vi "Update DO Bit with Index_PrivateData.vi"(8 "error in (no error)":errorcluster, 9 "Value":bool, 10 "index":i32, 11 "IO in":refnum<class "IO.lvclass">) -> (0 "error out":errorcluster, 2 "DO Bits Value":bool[](array[boolean]), 3 "IO out":refnum<class "IO.lvclass">)   [LabVIEW 2022 SP3, in "IO.lvclass"]
uses:
  IO.lvclass
  IO.lvclass/IO.ctl
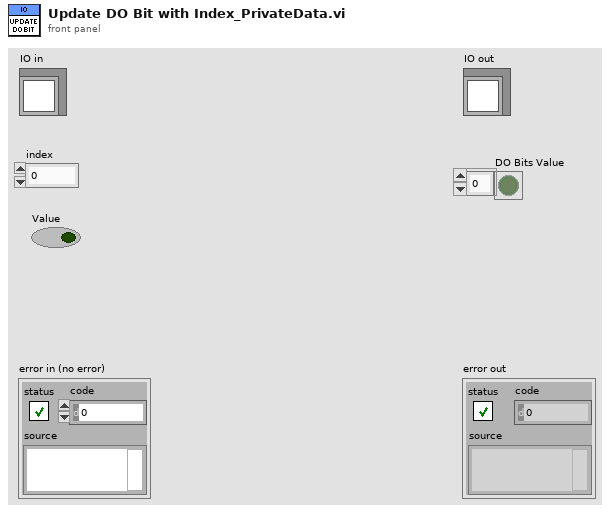
[diagram p1: front panel]
types:
  T1 = typedef "IO.lvclass/Private Data.ctl" = cluster{"UserEvents":T2, "All Dependencies":cluster{"Class References":refnum<class>[], "Class Names":string[]}, "Status":T3}
  T2 = typedef "IO.lvclass/UserEvents.ctl" = cluster{"API Incoming Event":refnum<user-event>, "API Executed Event":refnum<user-event>, "API Return Event":refnum<user-event>, "Status Changed Event":refnum<user-event>}
  T3 = typedef "IO.lvclass/Status Cluster.ctl" = cluster{"DO Bits Value":bool[], "Device Data":variant, "Ordered DI Channels":T4[], "Ordered DO Channels":T5[]}
  T4 = typedef "IO.lvclass/DI Channel Names.ctl" = enum16{"None", "SW - Ink Valve - R1", "SW - Ink Valve - R2", "SW - Ink Valve - R3", "SW - Ink Valve - R4", "SW - Ink Valve - R5", "SW - Ink Valve - R6", "SW - COVER INPUT SIDE", "SW - COVER OUTPUT SIDE", "SW - Purge - R1", "SW - Purge - R2", "SW - Purge - R3", "SW - Purge - R4", "SW - Purge - R5", "SW - Purge - R6"}
  T5 = typedef "IO.lvclass/DO Channel Names.ctl" = enum16{"None", "Meniscus Valve Open - R1", "Meniscus Valve Open - R2", "Meniscus Valve Open - R3", "Meniscus Valve Open - R4", "Meniscus Valve Open - R5", "Meniscus Valve Open - R6", "Ink Flow Valve Open - R1", "Ink Flow Valve Open - R2", "Ink Flow Valve Open - R3", "Ink Flow Valve Open - R4", "Ink Flow Valve Open - R5", "Ink Flow Valve Open - R6", "SW_LED - Ink Valve - R1", "SW_LED - Ink Valve - R2", "SW_LED - Ink Valve - R3", "Recirc Pump On - R1", "Recirc Pump On - R2", "Recirc Pump On - R3", "Recirc Pump On - R4", "Recirc Pump On - R5", "Recirc Pump On - R6", "SW_LED - Ink Valve - R4", "SW_LED - Ink Valve - R5", "SW_LED - Ink Valve - R6"}
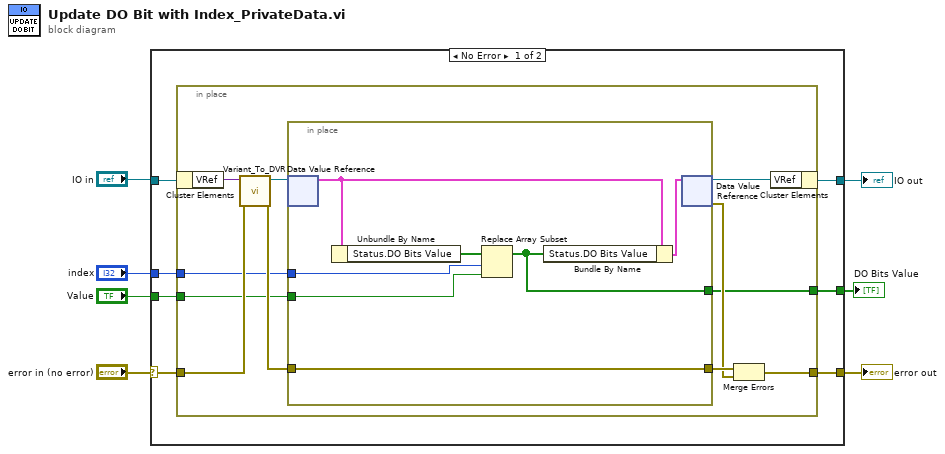
[diagram p0: block diagram]
diagram:
  n1 = case shown="No Error" "error in (no error)" {
    selector: "error in (no error)" -> [w11 w34]
    tunnel: [w13 w34] -> w5
    tunnel: [w14 w33] -> w4
    tunnel: "IO in" -> [w12 w33]
    tunnel: "index" -> [w10 _]
    tunnel: "Value" -> [w9 _]
    tunnel: [w8 _] -> w1
    frame No Error {
      n2 = in-place {
        in-place-border: w11 -> [w23]
        in-place-border: [w19] -> w13
        in-place-border: w10 -> [w17]
        in-place-border: w9 -> [w16]
        in-place-border: [w15] -> w8
        n3 = in-place-cluster #1(w12) -> ("VRef"=w25:variant)
        n4 = call "Variant_To_DVR.vi"("error in (no error)"=w23, "Variant"=w25) -> ("error out"=w22:errorcluster, "DVR"=w24:refnum<data-value>)  [unwired: 8 in]
        n5 = in-place {
          in-place-border: w22 -> [w32]
          in-place-border: [w32] -> w21
          in-place-border: w17 -> [w28]
          in-place-border: w16 -> [w27]
          in-place-border: [w26] -> w15
          n6 = in-place-dvr #2(w24) -> (w30:T1)  [unwired: 1 out]
          n7 = Unbundle By Name(w30) -> ("Status.DO Bits Value"=w31:bool[])
          n8 = Replace Array Subset(array=w31, new element=w27, index=w28) -> (w26:bool[])
          n9 = Bundle By Name(cluster=w30, "Status.DO Bits Value"=w26) -> (w29:T1)
          n10 = in-place-dvr #2(w29) -> (w18:refnum<data-value>, w20:errorcluster)
        }
        n11 = Merge Errors(w21, w20) -> (w19:errorcluster)
        n12 = in-place-cluster #1("VRef"=w18) -> (w14:refnum<class "IO.lvclass">)
      }
    }
    frame Error {
    }
  }
  "error out" <- w5
  "IO out" <- w4
  "DO Bits Value" <- w1
